vi "DAQSIM.vi"() -> ()   [LabVIEW 2021]
panel:
  in  "Stop":bool
  out "data":dynamicdata(graph)
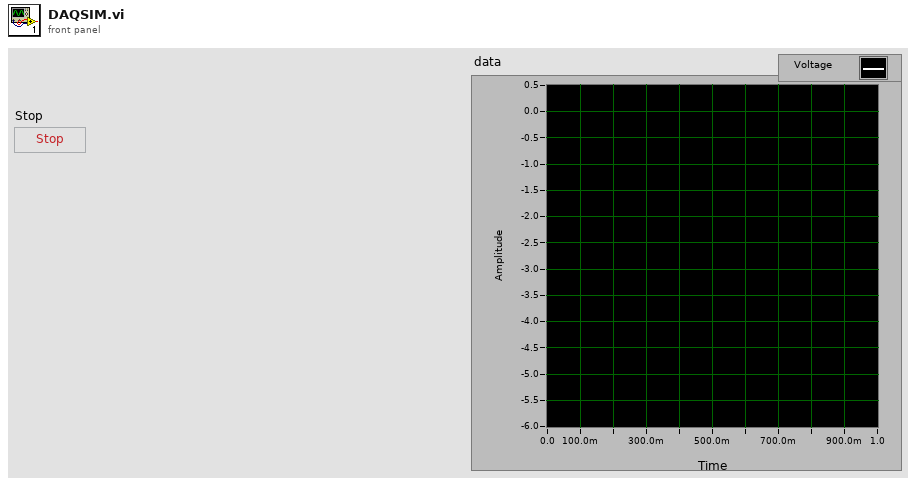
[diagram p1: front panel]
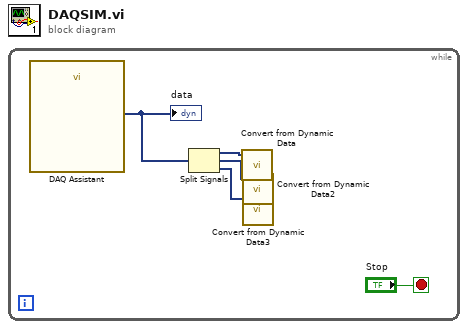
[diagram p0: block diagram]
diagram:
  n1 = while {
    stop <- "Stop" stop-if-true
    n2 = call "DAQ Assistant"() -> ("data"=w4:dynamicdata)  [unwired: 17 in, 2 out]
    "data" <- w4
    n3 = Split Signals(w4) -> (w3:dynamicdata, w2:dynamicdata, w1:dynamicdata)  [unwired: 3 in]
    n4 = call "Convert from Dynamic Data"("Dynamic Data Type"=w3) -> ()  [unwired: 3 in, 1 out]
    n5 = call "Convert from Dynamic Data2"("Dynamic Data Type"=w2) -> ()  [unwired: 3 in, 1 out]
    n6 = call "Convert from Dynamic Data3"("Dynamic Data Type"=w1) -> ()  [unwired: 3 in, 1 out]
  }
